vi "PRF_Set.vi"(6 "Location":T1, 8 "Motion Settings In":T2={"No Motion?"=FALSE, "Motion System"=enum."MM3000", "Motion Bd ID"=0, "Motion Profile"="", "# Axis"=0, "Reverse Z axis?"=FALSE, "SMAC Axis"=0, "scan pair"=enum."y-(x) scan", "RT fps"=0.0, "Steps per mm"=[], "Motor Parameters"={"velocity ct/s"=[], "accel ct/s^2"=[]}, "One Way Scan"=FALSE, "Reverse One Way Scan"=FALSE, "Global Position (mm)"=[], "Plane"=0, "Distance between\nscan lines (um)"=0.0, "Distance between\nscan planes (um)"=0.0, "number of scan planes"=0, "Total steps in line"=0, "Xtra plane\ndistance  (um)"=0, "Xtra planes "=0, "Add Axis"=FALSE, "overshoot cts"=0, "BKPT Shift"=0, "Scan Start Time (ms)"=0, "ESP VISA"="", "3rd Axis"=1, "GL Ref Out"=refnum, "Galil Address"=""} {"3rd Axis" items=["x", "y", "z", "w"]; "Xtra planes" min=1; "Xtra plane\ndistance  (um)" min=0; "Distance between\nscan planes (um)" format="%.2f"; "Distance between\nscan lines (um)" format="%.2f"; "SMAC Axis" items=["None"=0, "Axis 1"=1, "Axis 2"=2, "Axis 3"=3, "Axis 4"=4, "Axis 5"=5, "Axis 6"=6, "Axis 7"=7, "Axis 8"=8, "Vector Space 1"=17, "Vector Space 2"=18, "Vector Space 3"=19, "Vector Space 4"=20]; "Motion Bd ID" min=1 max=32 step=1}, 9 "prf (kHz)":dbl, 10 "Multi Trig?":bool, 11 "CTR PRF?":bool) -> ()   [LabVIEW 2022 SP3]
uses:
  Motion Controllers/NI_controller/-NI_MotionRoutines/MotionParameters.ctl
  Motion Controllers/NI_controller/-NI_MotionRoutines/MotionSys.ctl
  Motion Controllers/-MotionRoutines/ScanAxis.ctl
  Motion Controllers/-MotionRoutines/3rdAxis.ctl
  Controls/location.ctl
  Motion Controllers/Galil/Command Menu.ctl
  <vilib>/DAQmx/create/channels.llb/DAQmx Create Channel (CO-Pulse Generation-Frequency).vi
  <vilib>/DAQmx/configure/timing.llb/DAQmx Timing (Implicit).vi
  Motion Controllers/-MotionRoutines/MotionGlobals.vi
  <instrlib>/Newport ESP301/Newport ESP301.lvlib
panel:
  # "1-D and 2-D B scan settings"
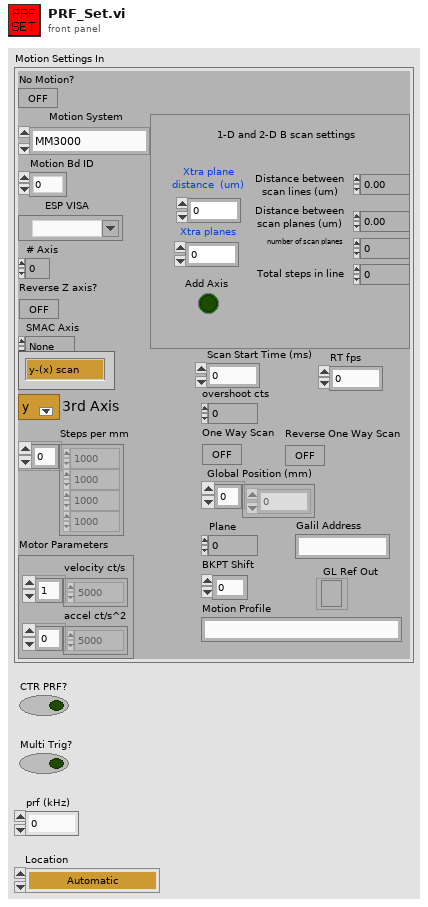
[diagram p1: front panel]
types:
  T1 = typedef "location.ctl" = enum16{"Automatic", "WCM Main", "Hawaii", "Columbia MM3000", "Columbia  NI System", "NYU", "RRI 2", "UHI Allen", "CUMC RT", "Chiba", "Stony Brook", "WCM Microscopy", "WCM Aeoretch", "WCM Optics Lab", "WCM Main 2Axis", "WCM Rotation", "WCM SAM SMAC", "SERI GP"}
  T2 = typedef "MotionParameters.ctl" = cluster{"No Motion?":bool, "Motion System":T3, "Motion Bd ID":u8, "Motion Profile":string, "# Axis":i8, "Reverse Z axis?":bool, "SMAC Axis":u16, "scan pair":T4, "RT fps":sgl, "Steps per mm":i32[], "Motor Parameters":cluster{"velocity ct/s":dbl[], "accel ct/s^2":dbl[]}, "One Way Scan":bool, "Reverse One Way Scan":bool, "Global Position (mm)":dbl[], "Plane":i32, "Distance between\nscan lines (um)":sgl, "Distance between\nscan planes (um)":sgl, "number of scan planes":i32, "Total steps in line":i32, "Xtra plane\ndistance  (um)":i32, "Xtra planes ":i32, "Add Axis":bool, "overshoot cts":i32, "BKPT Shift":i32, "Scan Start Time (ms)":u32, "ESP VISA":refnum<visa-resource-name>, "3rd Axis":T5, "GL Ref Out":refnum<k7>, "Galil Address":string}
  T3 = typedef "MotionSys.ctl" = enum16{"MM3000", "NI 735x", "Newport ESP", "No Motion Card", "Galil"}
  T4 = typedef "ScanAxis.ctl" = enum16{"y-(x) scan", "x-(y) scan", "z-(x) scan", "z-(y) scan", "y-(z) scan", "x-(z) scan", "w-(x) scan", "w-(y) scan", "w-(z) scan", "x-(w) scan", "y-(w) scan", "z-(w) scan"}
  T5 = typedef "3rdAxis.ctl" = u16
  T6 = typedef "Command Menu.ctl" = enum16{"CommandPassThrough", "Abort Motion", "Define Pos", "Velocity", "Acceleration", "Deceleration", "Position Rel", "Postion Abs", "Begin Move", "After Move", "Home", "KI", "KD", "KP", "IL", "Config I/O", "Set Bit", "Clear Bit", "Motor Off", "Moto On", "Status", "Execute", "Halt Execute", "HX Status", "Tell Velocity", "Check Motion", "BreakPoint", "Tell Position", "Current Code Line", "Tell Switches", "OC Force On", "OC Off", "Pos Soft Limit", "Rev Soft Limit"}
  T7 = cluster{"Port A bit-0 at logic level":bool, "Port A bit-1 at logic level":bool, "Port A bit-2 at logic level ":bool, "Port A bit-3 at logic level":bool, "Port A bit-4 at logic level":bool, "Port A bit-5 at logic level ":bool, "Port A bit-6 at logic level ":bool, "Port A bit-7 at logic level ":bool, "Port B bit-0 at logic level":bool, "Port B bit-1 at logic level":bool, "Port B bit-2 at logic level ":bool, "Port B bit-3 at logic level":bool, "Port B bit-4 at logic level":bool, "Port B bit-5 at logic level ":bool, "Port B bit-6 at logic level ":bool, "Port B bit-7 at logic level ":bool}
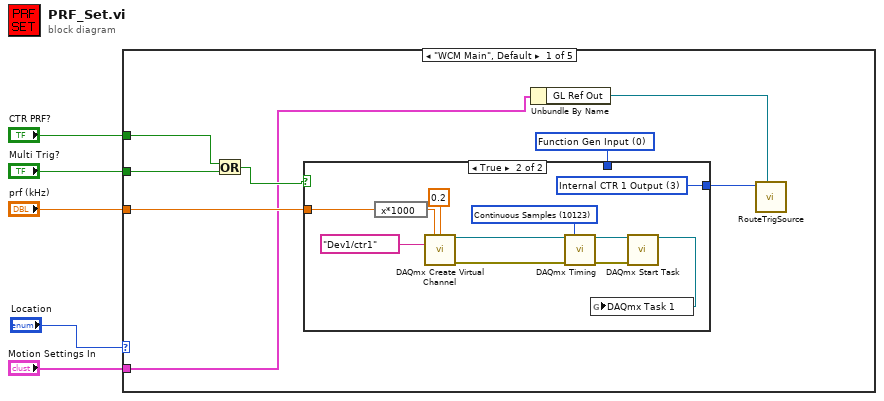
[diagram p0: block diagram]
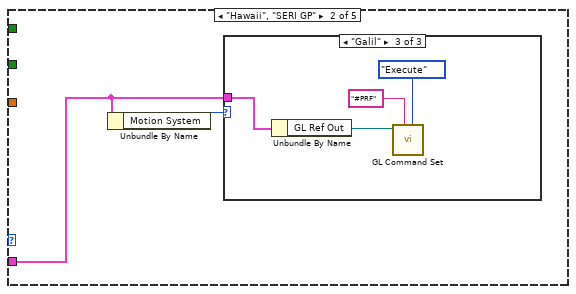
[diagram p3: hidden frame]
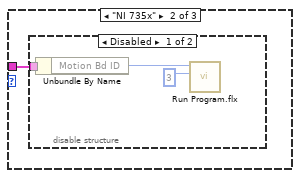
[diagram p5: hidden frame]
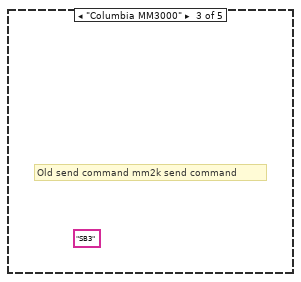
[diagram p7: hidden frame]
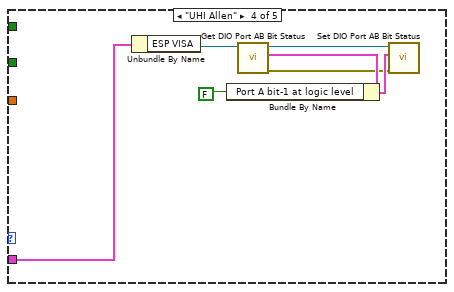
[diagram p8: hidden frame]
diagram:
  n1 = case shown="\"WCM Main\", Default" "Location" {
    tunnel: "prf (kHz)" -> [w12 _ _ _ _]
    tunnel: "CTR PRF?" -> [w11 _ _ _ _]
    tunnel: "Multi Trig?" -> [w10 _ _ _ _]
    tunnel: "Motion Settings In" -> [w7 w27 _ w37 _]
    frame "WCM Main", Default {
      w9 = u16 0 items=["Function Gen Input", "Motion Trig", "Internal RT Motion Trig", "Internal CTR 1 Output"] ("Trig Source")
      n2 = Or(x=w11, y=w10) -> (x .or. y?=w13:bool)
      n3 = case shown="True" w13 {
        tunnel: w12 -> [_ w20]
        tunnel: [w14 w15] -> w8
        tunnel: w9 -> [w14 _]
        frame False {
        }
        frame True {
          w15 = u16 3 items=["Function Gen Input", "Motion Trig", "Internal RT Motion Trig", "Internal CTR 1 Output"] ("Trig Source")
          w22 = 10123 items=["Finite Samples"=10178, "Continuous Samples"=10123, "Hardware Timed Single Point"=12522] ("sample mode")
          n4 = expression code="x*1000"(w20) -> (w21:dbl)
          n5 = call-poly <vilib>:"DAQmx Create Virtual Channel.vi"("frequency"=w21, "duty cycle"=0.2, "counter"=tag "Dev1/ctr1") -> ("task out"=w24:refnum<k21>, "error out"=w23:errorcluster)  [unwired: 6 in, 5 out]
          n6 = call-poly <vilib>:"DAQmx Timing.vi"("task/channels in"=w24, "sample mode"=w22, "error in"=w23) -> ("task out"=w18:refnum<k21>, "error out"=w17:errorcluster)  [unwired: 11 in]
          n7 = call <vilib>:"DAQmx Start Task.vi"("task/channels in"=w18, "error in"=w17) -> ("task out"=w16:refnum<k21>)  [unwired: 12 in, 1 out]
          n8 = global write "MotionGlobals.vi" "DAQmx Task 1"(w16) -> ()
        }
      }
      n9 = Unbundle By Name(w7) -> ("GL Ref Out"=w6:refnum<k7>)
      n10 = call "RouteTrigSource.vi"("Galil.IGalil"=w6, "Trig Source"=w8) -> ()  [unwired: 9 in, 1 out]
    }
    frame "Hawaii", "SERI GP" {
      n11 = Unbundle By Name(w27) -> ("Motion System"=w26:T3)
      n12 = case shown="\"Galil\"" w26 {
        tunnel: w27 -> [_ w28 w35]
        frame "MM3000", Default {
        }
        frame "NI 735x" {
          n13 = disable-structure shown="Disabled" {
            disable-tunnel: w28 -> [w29 _]
            frame Disabled {
              n14 = Unbundle By Name(w29) -> ("Motion Bd ID"=w30:u8)
              n15 = call <vilib>:"Run Program.flx"("Program (1)"=3, "Board ID"=w30) -> ()  [unwired: 1 in, 6 out]
            }
            frame Enabled {
            }
          }
        }
        frame "Galil" {
          n16 = Unbundle By Name(w35) -> ("GL Ref Out"=w34:refnum<k7>)
          n17 = call "GL Command Set.vi"("Command"=Command_Menu."Execute", "Text Input"="#PRF", "Galil.IGalil"=w34) -> ()  [unwired: 4 in, 5 out]
        }
      }
    }
    frame "Columbia MM3000" {
      (unwired) "SB3"
      # "Old send command mm2k send command"
    }
    frame "UHI Allen" {
      n18 = Unbundle By Name(w37) -> ("ESP VISA"=w36:refnum<visa-resource-name>)
      n19 = call <instrlib>:"Get DIO Port AB Bit Status.vi"("VISA resource name"=w36) -> ("error out"=w39:errorcluster, "DIO Port A status"=w42:T7, "VISA resource name out"=w38:refnum<visa-resource-name>)  [unwired: 4 in]
      n20 = Bundle By Name(cluster=w42, "Port A bit-1 at logic level"=FALSE) -> (w40:T7)
      n21 = call <instrlib>:"Set DIO Port AB Bit Status.vi"("error in (no error)"=w39, "DIO Port status"=w40, "VISA resource name"=w38) -> ()  [unwired: 3 in, 2 out]
    }
    frame "CUMC RT" {
    }
  }
